vi "基础 1.vi"(8 "转盘":dbl(knob) scale=0.0..10.0, 9 "布尔":bool=TRUE, 11 "旋钮":dbl(knob) scale=0.0..10.0) -> (4 "波形图":waveform(dbl)(graph))   [LabVIEW 2014]
uses:
  <vilib>/measure/NI_MABase.lvlib
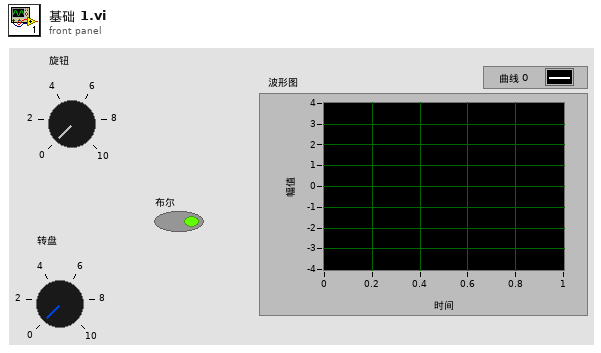
[diagram p1: front panel]
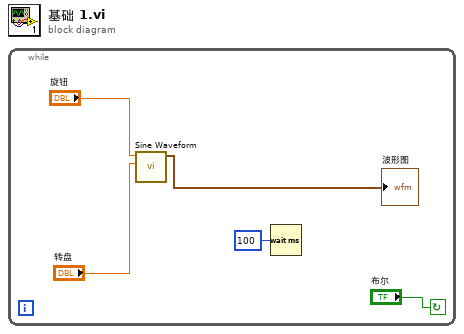
[diagram p0: block diagram]
diagram:
  n1 = while {
    stop <- "布尔" continue-if-true
    n2 = call <vilib>:"Sine Waveform.vi"("amplitude"="转盘", "frequency"="旋钮") -> ("signal out"=→"波形图":waveform(dbl))  [unwired: 8 in, 1 out]
    n3 = Wait (ms)(milliseconds to wait=u32 100 ("等待时间（毫秒）")) -> ()  [unwired: 1 out]
  }
